vi "Drive_Hardware_Begin.vi"(8 "error in":errorcluster) -> (0 "error out":errorcluster)   [LabVIEW 2020]
uses:
  <vilib>/Rock Robotics/WPI/ThirdParty/Phoenix-LabVIEW/Motor Controller/Controls/CTRE_Phoenix_MotorControl_BaseConfigurables.ctl
  <vilib>/Rock Robotics/WPI/ThirdParty/Phoenix-LabVIEW/Motor Controller/Controls/CTRE_Phoenix_MotorControl_VelocityMeasurementPeriod.ctl
  <vilib>/Rock Robotics/WPI/ThirdParty/Phoenix-LabVIEW/Motor Controller/Controls/CTRE_Phoenix_MotorControl_SlotStructure.ctl
  <vilib>/Rock Robotics/WPI/ThirdParty/Phoenix-LabVIEW/Motor Controller/Controls/CTRE_Phoenix_MotorControl_FilterStruct.ctl
  <vilib>/Rock Robotics/WPI/ThirdParty/Phoenix-LabVIEW/Motor Controller/Controls/CTRE_Phoenix_MotorControl_RemoteSourceType.ctl
  <vilib>/Rock Robotics/WPI/ThirdParty/Phoenix-LabVIEW/Controls/CTRE_Phoenix_CustomParamConfiguration.ctl
  <vilib>/Rock Robotics/WPI/ThirdParty/Phoenix-LabVIEW/Motor Controller/Controls/CTRE_Phoenix_MotorControl_FeedbackDevice_TalonFX.ctl
  <vilib>/Rock Robotics/WPI/ThirdParty/Phoenix-LabVIEW/Motor Controller/Controls/CTRE_Phoenix_MotorControl_LimitSwitchNormal.ctl
  <vilib>/Rock Robotics/WPI/ThirdParty/Phoenix-LabVIEW/Motor Controller/Controls/CTRE_Phoenix_MotorControl_LimitSwitchSource_Local.ctl
  <vilib>/Rock Robotics/WPI/ThirdParty/Phoenix-LabVIEW/Motor Controller/Controls/CTRE_Phoenix_MotorControl_SupplyCurrentLimitConfiguration.ctl
  <vilib>/Rock Robotics/WPI/ThirdParty/Phoenix-LabVIEW/Motor Controller/Controls/CTRE_Phoenix_MotorControl_StatorCurrentLimitConfiguration.ctl
  <vilib>/Rock Robotics/WPI/ThirdParty/Phoenix-LabVIEW/Motor Controller/Controls/CTRE_Phoenix_MotorControl_MotorCommutation_TalonFX.ctl
  <vilib>/Rock Robotics/WPI/ThirdParty/Phoenix-LabVIEW/CANCoder/Controls/CTRE_Phoenix_CANcoder_AbsoluteSensorRange.ctl
  <vilib>/Rock Robotics/WPI/ThirdParty/Phoenix-LabVIEW/CANCoder/Controls/CTRE_Phoenix_CANcoder_SensorInitializationStrategy.ctl
  <vilib>/Rock Robotics/WPI/ThirdParty/Phoenix-LabVIEW/Motor Controller/Controls/CTRE_Phoenix_MotorControl_TalonFXInvertType.ctl
  <vilib>/Rock Robotics/WPI/ThirdParty/Phoenix-LabVIEW/Motor Controller/Controls/CTRE_Phoenix_MotorControl_NeutralMode.ctl
  <vilib>/Rock Robotics/WPI/ThirdParty/Phoenix-LabVIEW/CANCoder/Controls/CTRE_Phoenix_CANcoder_StatusFrame.ctl
  <vilib>/Rock Robotics/WPI/ThirdParty/Phoenix-LabVIEW/Pigeon IMU/CTRE_PigeonIMU_StatusFrameRate.ctl
  Drive_Hardware_Globals.vi
  Globals/Status_Frame_Rate_Globals.vi
  Globals/FilePath_Globals.vi
  Globals/Calibration_And_Constant_Globals.vi
  <vilib>/Utility/file.llb/Read Delimited Spreadsheet (DBL).vi
  Globals/Drive_Globals.vi
panel:
  in  "Front_Right_Zero":dbl[](array[numeric])=[99.4, 331.43]
  in  "Front_Left_Zero":dbl[](array[numeric])=[338.818, 288.54]
  in  "Back_Left_Zero":dbl[](array[numeric])=[255.059, 271.84]
  in  "Back_Right_Zero":dbl[](array[numeric])=[182.197, 189.4]
  out "elements":i32
  out "File Read Error":bool
  out "appended path":path
  in  "Talon FX Configurables":T15={"Base Configurables"={"openLoopRamp"=0.0, "closedLoopRamp"=0.0, "peakOutputForward"=1.0, "peakOutputReverse"=-1.0, "nominalOutputForward"=0.0, "nominalOutputReverse"=0.0, "neutralDeadband"=0.0, "voltageCompSaturation"=0.0, "voltageMeasurementFilter"=32, "velocityMeasurementPeriod"=100, "velocityMeasurementWindow"=64, "forwardSoftLimitThreshold"=0, "reverseSoftLimitThreshold"=0, "forwardSoftLimitEnable"=FALSE, "reverseSoftLimitEnable"=FALSE, "slot0"={"P"=0.0, "I"=0.0, "D"=0.0, "F"=0.0, "integralZone"=0.0, "allowableClosedLoopError"=0, "maxIntegralAccumulator"=0.0, "closedLoopPeakOutput"=1.0, "closedLoopPeriod"=1}, "slot1"={"P"=0.0, "I"=0.0, "D"=0.0, "F"=0.0, "integralZone"=0.0, "allowableClosedLoopError"=0, "maxIntegralAccumulator"=0.0, "closedLoopPeakOutput"=1.0, "closedLoopPeriod"=1}, "slot2"={"P"=0.0, "I"=0.0, "D"=0.0, "F"=0.0, "integralZone"=0.0, "allowableClosedLoopError"=0, "maxIntegralAccumulator"=0.0, "closedLoopPeakOutput"=1.0, "closedLoopPeriod"=1}, "slot3"={"P"=0.0, "I"=0.0, "D"=0.0, "F"=0.0, "integralZone"=0.0, "allowableClosedLoopError"=0, "maxIntegralAccumulator"=0.0, "closedLoopPeakOutput"=1.0, "closedLoopPeriod"=1}, "auxPIDPolarity"=FALSE, "remoteFilter0"={"remoteSensorDeviceID"=0, "remoteSensorSource"=enum."Off"}, "remoteFilter1"={"remoteSensorDeviceID"=0, "remoteSensorSource"=enum."Off"}, "motionCruiseVelocity"=0, "motionAcceleration"=0, "motionProfileTrajectoryPeriod"=0, "feedbackNotContinuous"=FALSE, "remoteSensorClosedLoopDisableNeutralOnLOS"=FALSE, "clearPositionOnLimitF"=FALSE, "clearPositionOnLimitR"=FALSE, "clearPositionOnQuadIdx"=FALSE, "limitSwitchDisableNeutralOnLOS"=FALSE, "softLimitDisableNeutralOnLOS"=FALSE, "pulseWidthPeriod_EdgesPerRot"=1, "pulseWidthPeriod_FilterWindowSz"=1, "customParam"={"customParam0"=0, "customParam1"=0}, "trajectoryInterpolationEnable"=TRUE}, "primaryPID"={"selectedFeedbackCoefficient"=1.0, "selectedFeedbackSensor"=1}, "auxiliaryPID"={"selectedFeedbackCoefficient"=1.0, "selectedFeedbackSensor"=1}, "forwardLimitSwitchNormal"=enum."Normally Open", "reverseLimitSwitchNormal"=enum."Normally Open", "forwardLimitSwitchDeviceID"=0, "reverseLimitSwitchDeviceID"=0, "forwardLimitSwitchSource"=enum."Feedback Connector", "reverseLimitSwitchSource"=enum."Feedback Connector", "sum0Term"=1, "sum1Term"=1, "diff0Term"=1, "diff1Term"=1, "Supply Current Limit Configuration"={"Enable?"=FALSE, "Current Limit"=0.0, "Threshold Current"=0.0, "Threshold Time"=0.0}, "Stator Current Limit Configuration"={"Enable?"=FALSE, "Current Limit"=0.0, "Threshold Current"=0.0, "Threshold Time"=0.0}, "Motor Commutation"=enum."Trapezoidal", "Absolute Sensor Range"=enum."Unsigned [0 to 360)", "Integrated Sensor Offset (Degrees)"=0.0, "Sensor Initialization Strategy"=enum."Boot To Zero"} {"Base Configurables"."velocityMeasurementPeriod" items=["Period_1ms"=1, "Period_2ms"=2, "Period_5ms"=5, "Period_10ms"=10, "Period_20ms"=20, "Period_25ms"=25, "Period_50ms"=50, "Period_100ms"=100]; "primaryPID"."selectedFeedbackSensor" items=["Integrated Sensor"=1, "Sensor Sum (S0 + S1)"=9, "Sensor Difference (D0 - D1)"=10, "Remote Source 0"=11, "Remote Source 1"=12, "None"=14, "Software Emulated"=15]; "auxiliaryPID"."selectedFeedbackSensor" items=["Integrated Sensor"=1, "Sensor Sum (S0 + S1)"=9, "Sensor Difference (D0 - D1)"=10, "Remote Source 0"=11, "Remote Source 1"=12, "None"=14, "Software Emulated"=15]; "sum0Term" items=["Integrated Sensor"=1, "Sensor Sum (S0 + S1)"=9, "Sensor Difference (D0 - D1)"=10, "Remote Source 0"=11, "Remote Source 1"=12, "None"=14, "Software Emulated"=15]; "sum1Term" items=["Integrated Sensor"=1, "Sensor Sum (S0 + S1)"=9, "Sensor Difference (D0 - D1)"=10, "Remote Source 0"=11, "Remote Source 1"=12, "None"=14, "Software Emulated"=15]; "diff0Term" items=["Integrated Sensor"=1, "Sensor Sum (S0 + S1)"=9, "Sensor Difference (D0 - D1)"=10, "Remote Source 0"=11, "Remote Source 1"=12, "None"=14, "Software Emulated"=15]; "diff1Term" items=["Integrated Sensor"=1, "Sensor Sum (S0 + S1)"=9, "Sensor Difference (D0 - D1)"=10, "Remote Source 0"=11, "Remote Source 1"=12, "None"=14, "Software Emulated"=15]}
  # "0th index is alpha, 1st index is beta"
  # "False: Primary Output = PID[0] + PID[1]  ---  Auxiliary Output = PID[0] - PID[1]\nTrue:  Primary Output = PID[0] - PID[1] --- Auxiliary Output = PID[0] + PID[1]"
  # "Enable the motion profile executor to perform linear interpolation between profile points.  Defaults to True."
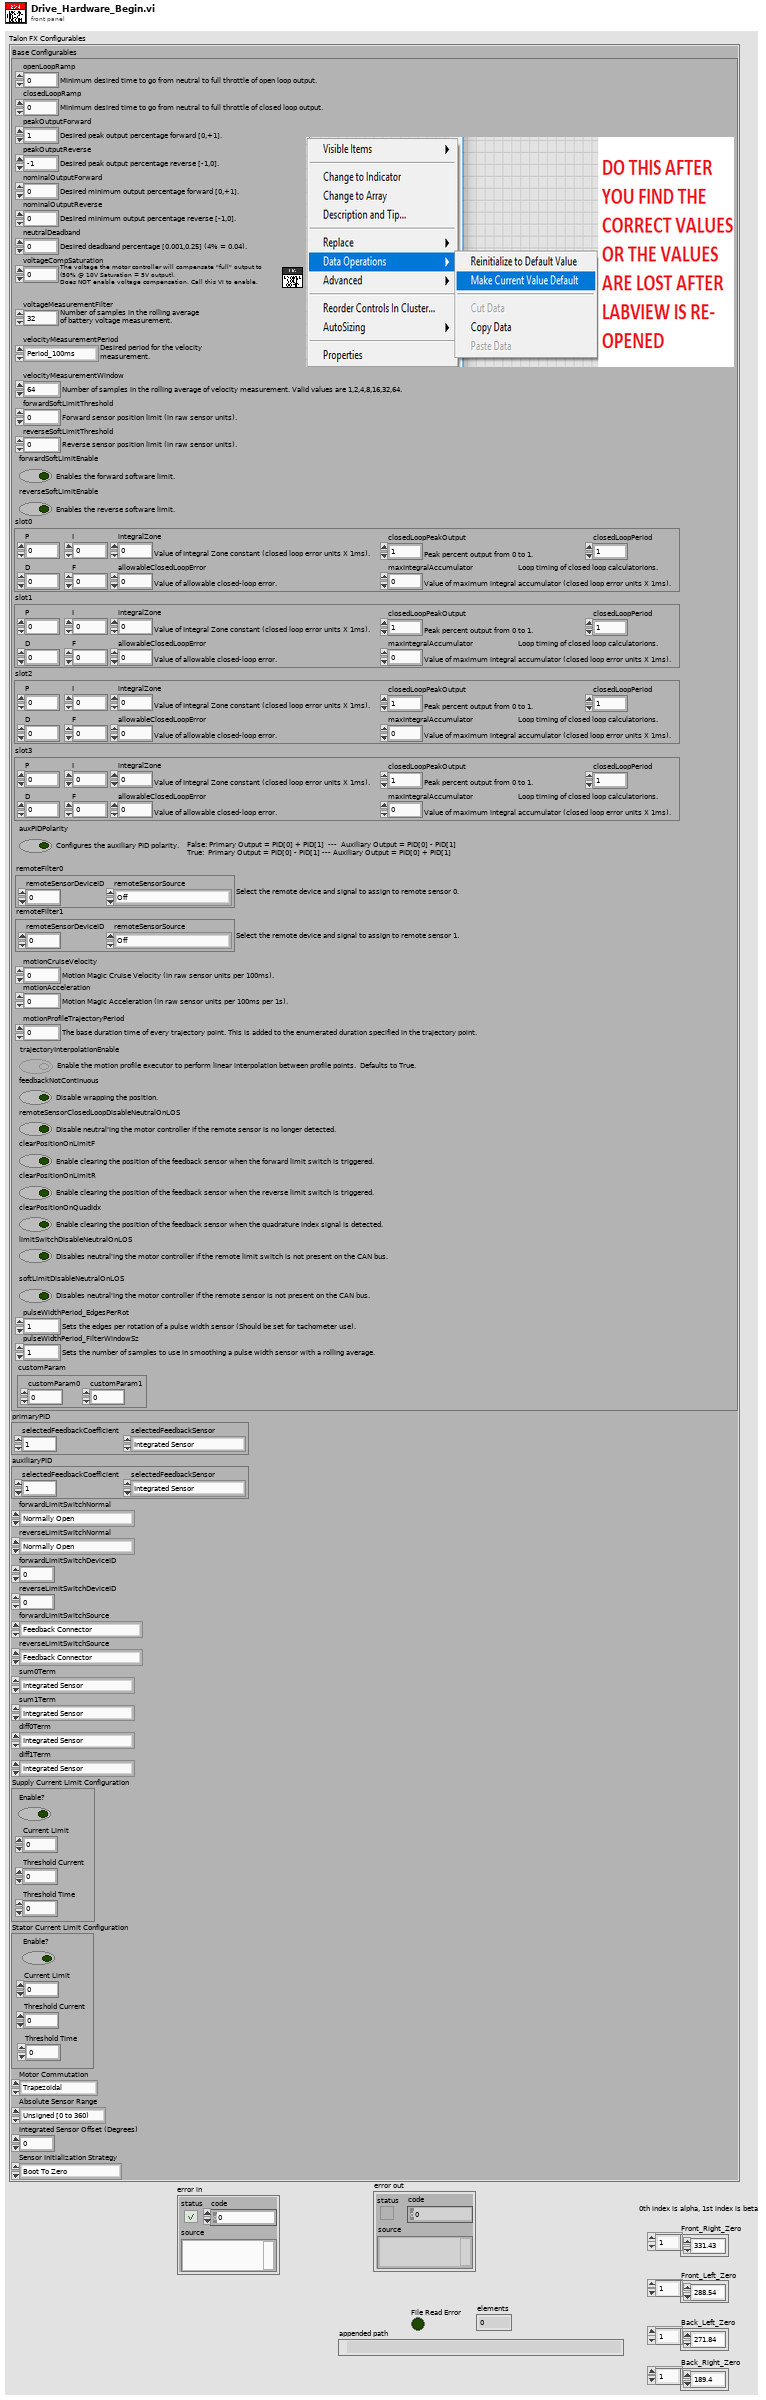
[diagram p1: front panel]
types:
  T1 = typedef "CTRE_Phoenix_MotorControl_BaseConfigurables.ctl" = cluster{"openLoopRamp":dbl, "closedLoopRamp":dbl, "peakOutputForward":dbl, "peakOutputReverse":dbl, "nominalOutputForward":dbl, "nominalOutputReverse":dbl, "neutralDeadband":dbl, "voltageCompSaturation":dbl, "voltageMeasurementFilter":i32, "velocityMeasurementPeriod":T2, "velocityMeasurementWindow":i32, "forwardSoftLimitThreshold":i32, "reverseSoftLimitThreshold":i32, "forwardSoftLimitEnable":bool, "reverseSoftLimitEnable":bool, "slot0":T3, "slot1":T3, "slot2":T3, "slot3":T3, "auxPIDPolarity":bool, "remoteFilter0":T4, "remoteFilter1":T4, "motionCruiseVelocity":i32, "motionAcceleration":i32, "motionProfileTrajectoryPeriod":i32, "feedbackNotContinuous":bool, "remoteSensorClosedLoopDisableNeutralOnLOS":bool, "clearPositionOnLimitF":bool, "clearPositionOnLimitR":bool, "clearPositionOnQuadIdx":bool, "limitSwitchDisableNeutralOnLOS":bool, "softLimitDisableNeutralOnLOS":bool, "pulseWidthPeriod_EdgesPerRot":i32, "pulseWidthPeriod_FilterWindowSz":i32, "customParam":T6, "trajectoryInterpolationEnable":bool}
  T2 = typedef "CTRE_Phoenix_MotorControl_VelocityMeasurementPeriod.ctl" = u16
  T3 = typedef "CTRE_Phoenix_MotorControl_SlotStructure.ctl" = cluster{"P":dbl, "I":dbl, "D":dbl, "F":dbl, "integralZone":dbl, "allowableClosedLoopError":i32, "maxIntegralAccumulator":dbl, "closedLoopPeakOutput":dbl, "closedLoopPeriod":i32}
  T4 = typedef "CTRE_Phoenix_MotorControl_FilterStruct.ctl" = cluster{"remoteSensorDeviceID":u8, "remoteSensorSource":T5}
  T5 = typedef "CTRE_Phoenix_MotorControl_RemoteSourceType.ctl" = enum16{"Off", "Talon SRX Selected Sensor", "Pigeon IMU Yaw", "Pigeon IMU Pitch", "Pigeon IMU Roll", "CANifier Quadrature", "CANifier PWM Input 0", "CANifier PWM Input 1", "CANifier PWM Input 2", "CANifier PWM Input 3", "Gadgeteer Pigeon Yaw", "Gadgeteer Pigeon Pitch", "Gadgeteer Pigeon Roll", "CANCoder"}
  T6 = typedef "CTRE_Phoenix_CustomParamConfiguration.ctl" = cluster{"customParam0":i32, "customParam1":i32}
  T7 = typedef "CTRE_Phoenix_MotorControl_FeedbackDevice_TalonFX.ctl" = i8
  T8 = typedef "CTRE_Phoenix_MotorControl_LimitSwitchNormal.ctl" = enum16{"Normally Open", "Normally Closed", "Disabled"}
  T9 = typedef "CTRE_Phoenix_MotorControl_LimitSwitchSource_Local.ctl" = enum16{"Feedback Connector", "Remote Talon SRX", "Remote CANifier", "Deactivated"}
  T10 = typedef "CTRE_Phoenix_MotorControl_SupplyCurrentLimitConfiguration.ctl" = cluster{"Enable?":bool, "Current Limit":dbl, "Threshold Current":dbl, "Threshold Time":dbl}
  T11 = typedef "CTRE_Phoenix_MotorControl_StatorCurrentLimitConfiguration.ctl" = cluster{"Enable?":bool, "Current Limit":dbl, "Threshold Current":dbl, "Threshold Time":dbl}
  T12 = typedef "CTRE_Phoenix_MotorControl_MotorCommutation_TalonFX.ctl" = enum16{"Trapezoidal"}
  T13 = typedef "CTRE_Phoenix_CANcoder_AbsoluteSensorRange.ctl" = enum16{"Unsigned [0 to 360)", "Signed [-180 to +180)"}
  T14 = typedef "CTRE_Phoenix_CANcoder_SensorInitializationStrategy.ctl" = enum16{"Boot To Zero", "Boot To Absolute Position"}
  T15 = cluster{"Base Configurables":T1, "primaryPID":cluster{"selectedFeedbackCoefficient":dbl, "selectedFeedbackSensor":T7}, "auxiliaryPID":cluster{"selectedFeedbackCoefficient":dbl, "selectedFeedbackSensor":T7}, "forwardLimitSwitchNormal":T8, "reverseLimitSwitchNormal":T8, "forwardLimitSwitchDeviceID":i32, "reverseLimitSwitchDeviceID":i32, "forwardLimitSwitchSource":T9, "reverseLimitSwitchSource":T9, "sum0Term":T7, "sum1Term":T7, "diff0Term":T7, "diff1Term":T7, "Supply Current Limit Configuration":T10, "Stator Current Limit Configuration":T11, "Motor Commutation":T12, "Absolute Sensor Range":T13, "Integrated Sensor Offset (Degrees)":dbl, "Sensor Initialization Strategy":T14}
  T16 = typedef "CTRE_PigeonIMU_StatusFrameRate.ctl" = u32
  T17 = typedef "CTRE_Phoenix_CANcoder_StatusFrame.ctl" = u32
  T18 = typedef "CTRE_Phoenix_MotorControl_TalonFXInvertType.ctl" = enum16{"Counter-Clockwise", "Clockwise"}
  T19 = typedef "CTRE_Phoenix_MotorControl_NeutralMode.ctl" = enum8{"EEPROMSetting", "Override to Coast", "Override to Brake"}
  T20 = typedef "WPI_MotorControlDeviceRef.ctl" = cluster{"DeviceStatus":errorcluster, "Type":T21, "PWM":cluster{"PWM Channel":T22, "DeadBand":T23}, "CAN":cluster{"Device Number":u8, "SetOutput VI Ref":variant, "GetOutput VI Ref":variant, "Enable VI Ref":variant, "Disable VI Ref":variant, "Data":variant}, "Invert":bool, "DIO PWM":cluster{"PWM \"Enable\" Channel":T22, "DIOChannel":T24, "PWM Rate":dbl}}
  T21 = typedef "WPI_MotorControlType.ctl" = enum16{"PWM", "CAN", "DIO PWM"}
  T22 = typedef "FPGA_DIOPWMChannel.ctl" = enum8{"PWM 0", "PWM 1", "PWM 2", "PWM 3", "PWM 4", "PWM 5", "PWM 6", "PWM 7", "PWM 8", "PWM 9", "PWM MXP 0", "PWM MXP 1", "PWM MXP 2", "PWM MXP 3", "PWM MXP 4", "PWM MXP 5", "PWM MXP 6", "PWM MXP 7", "PWM MXP 8", "PWM MXP 9", "Invalid"}
  T23 = typedef "WPI_PWMDeadband.ctl" = cluster{"Name":string, "maxPositivePwm":i32, "minPositivePwm":i32, "centerPwm":i32, "maxNegativePwm":i32, "minNegativePwm":i32, "angularRange":u16}
  T24 = typedef "FPGA_DIOChannel.ctl" = enum8{"DIO 0", "DIO 1", "DIO 2", "DIO 3", "DIO 4", "DIO 5", "DIO 6", "DIO 7", "DIO 8", "DIO 9", "DIO MXP 0", "DIO MXP 1", "DIO MXP 2", "DIO MXP 3", "DIO MXP 4", "DIO MXP 5", "DIO MXP 6", "DIO MXP 7", "DIO MXP 8", "DIO MXP 9", "DIO MXP 10", "DIO MXP 11", "DIO MXP 12", "DIO MXP 13", "DIO MXP 14", "DIO MXP 15", "SPI Port CS1", "SPI Port CS2", "SPI Port CS3", "SPI Port MISO", "SPI Port MOSI", "Invalid"}
  T25 = typedef "CTRE_PigeonIMU_DeviceRef.ctl" = cluster{"DeviceStatus":errorcluster, "Device Number":u8, "Type":T26, "Device ID":u32, "Handle":u64, "UsageFrame":u32, "Library Path":path}
  T26 = typedef "CTRE_PigeonIMU_ConnectionType.ctl" = u32
  T27 = typedef "CTRE_Phoenix_CANcoder_DeviceRef.ctl" = cluster{"DeviceStatus":errorcluster, "Device Number":u8, "Handle":u64, "UsageFrame":u32, "Library Path":path}
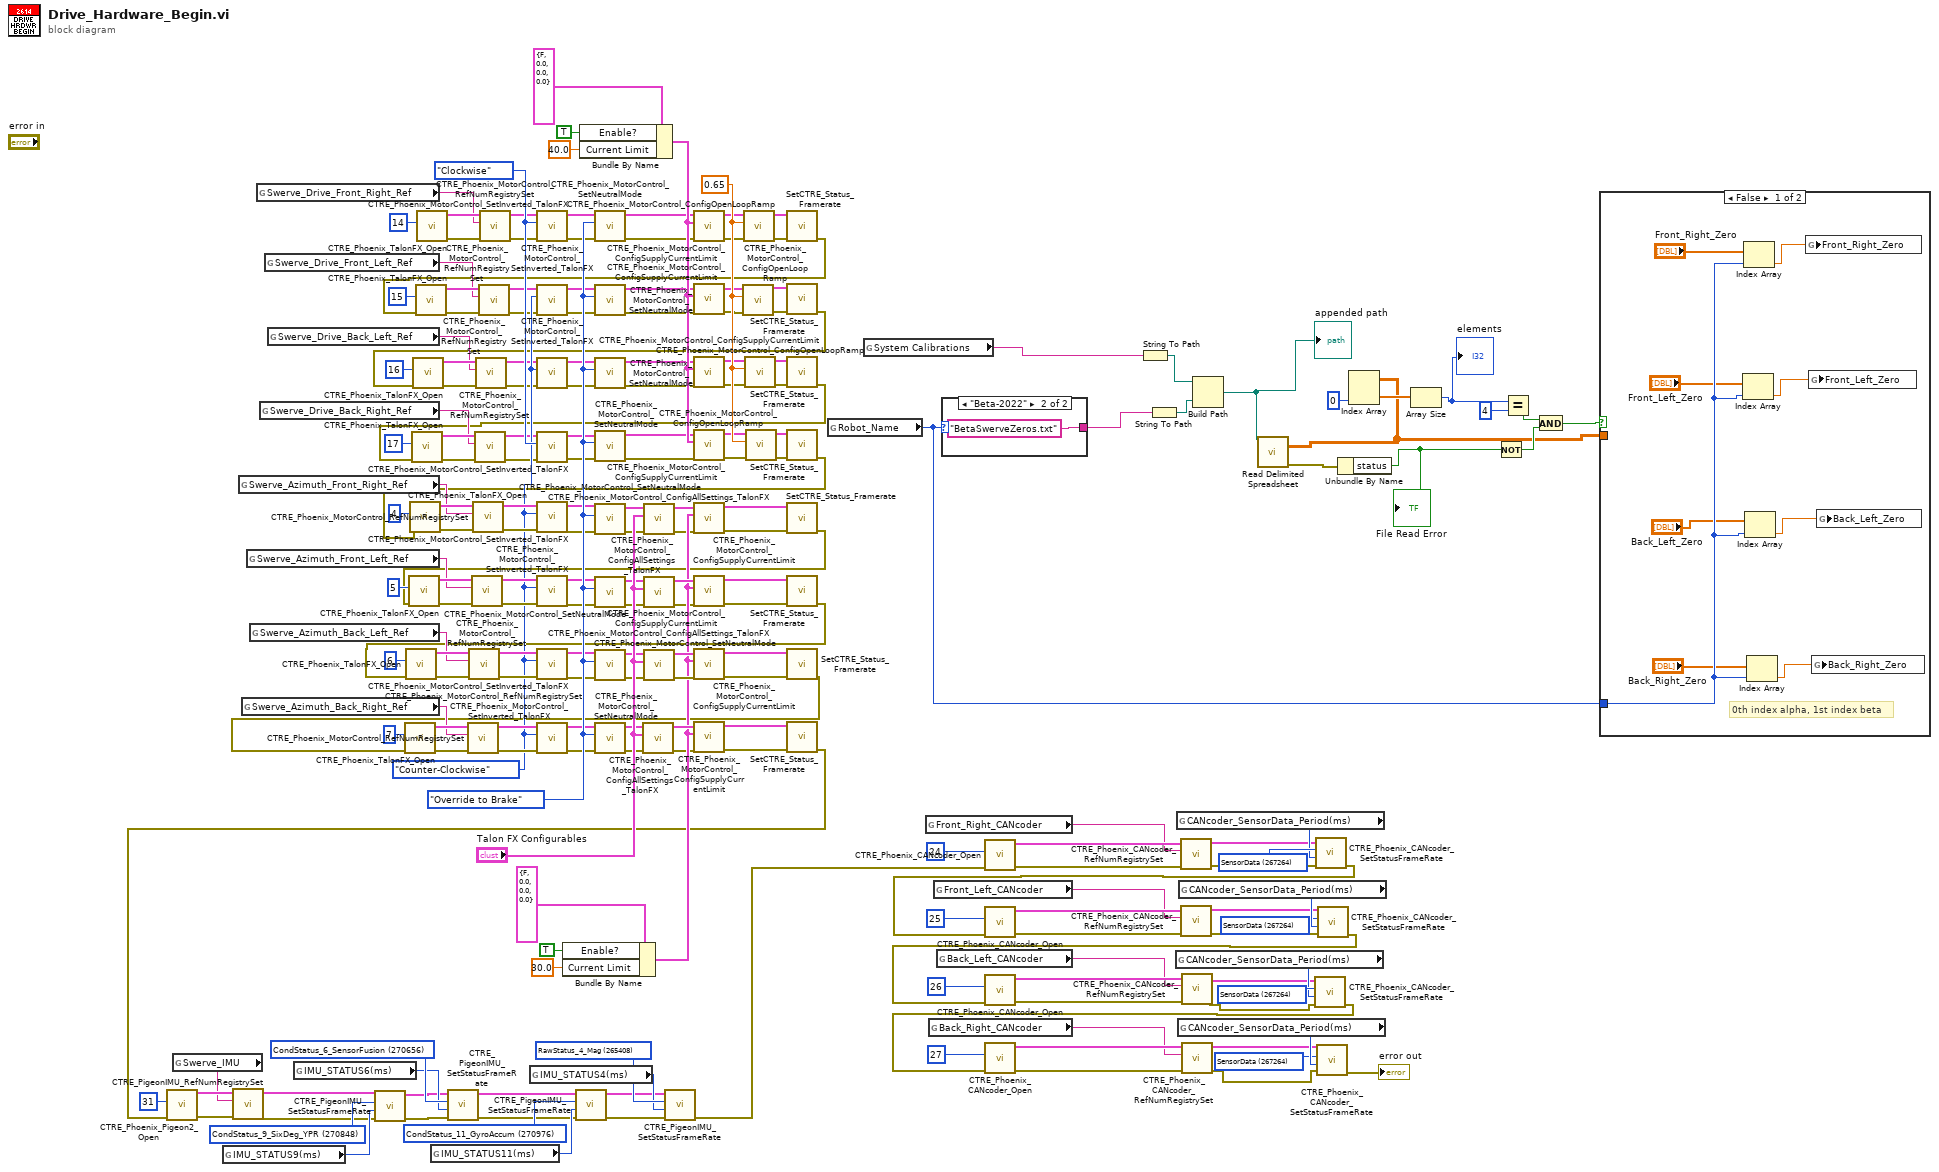
[diagram p0: block diagram]
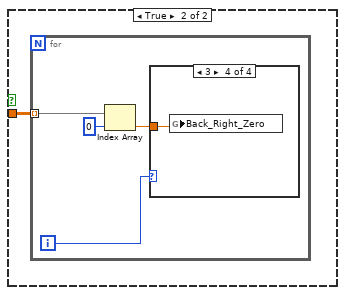
[diagram p2: hidden frame]
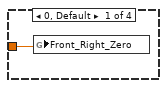
[diagram p3: hidden frame]
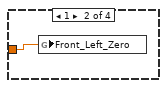
[diagram p4: hidden frame]
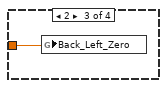
[diagram p5: hidden frame]
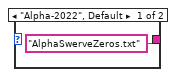
[diagram p6: hidden frame]
diagram:
  w31 = T16 265408 items=["CondStatus_1_General"=270336, "CondStatus_9_SixDeg_YPR"=270848, "CondStatus_6_SensorFusion"=270656, "CondStatus_11_GyroAccum"=270976, "CondStatus_2_GeneralCompass"=270400, "CondStatus_3_GeneralAccel"=270464, "CondStatus_10_SixDeg_Quat"=270912, "RawStatus_4_Mag"=265408, "BiasedStatus_2_Gyro"=269376, "BiasedStatus_4_Mag"=269504, "BiasedStatus_6_Accel"=269632] ("Pigeon IMU Status Frame")
  w32 = T16 270976 items=["CondStatus_1_General"=270336, "CondStatus_9_SixDeg_YPR"=270848, "CondStatus_6_SensorFusion"=270656, "CondStatus_11_GyroAccum"=270976, "CondStatus_2_GeneralCompass"=270400, "CondStatus_3_GeneralAccel"=270464, "CondStatus_10_SixDeg_Quat"=270912, "RawStatus_4_Mag"=265408, "BiasedStatus_2_Gyro"=269376, "BiasedStatus_4_Mag"=269504, "BiasedStatus_6_Accel"=269632] ("Pigeon IMU Status Frame")
  w33 = T16 270656 items=["CondStatus_1_General"=270336, "CondStatus_9_SixDeg_YPR"=270848, "CondStatus_6_SensorFusion"=270656, "CondStatus_11_GyroAccum"=270976, "CondStatus_2_GeneralCompass"=270400, "CondStatus_3_GeneralAccel"=270464, "CondStatus_10_SixDeg_Quat"=270912, "RawStatus_4_Mag"=265408, "BiasedStatus_2_Gyro"=269376, "BiasedStatus_4_Mag"=269504, "BiasedStatus_6_Accel"=269632] ("Pigeon IMU Status Frame")
  w34 = T16 270848 items=["CondStatus_1_General"=270336, "CondStatus_9_SixDeg_YPR"=270848, "CondStatus_6_SensorFusion"=270656, "CondStatus_11_GyroAccum"=270976, "CondStatus_2_GeneralCompass"=270400, "CondStatus_3_GeneralAccel"=270464, "CondStatus_10_SixDeg_Quat"=270912, "RawStatus_4_Mag"=265408, "BiasedStatus_2_Gyro"=269376, "BiasedStatus_4_Mag"=269504, "BiasedStatus_6_Accel"=269632] ("Pigeon IMU Status Frame")
  w45 = T17 267264 items=["SensorData"=267264, "VbatAndFaults"=267328] ("CANcoder Status Frame")
  w48 = T17 267264 items=["SensorData"=267264, "VbatAndFaults"=267328] ("CANcoder Status Frame")
  w49 = T17 267264 items=["SensorData"=267264, "VbatAndFaults"=267328] ("CANcoder Status Frame")
  w54 = T17 267264 items=["SensorData"=267264, "VbatAndFaults"=267328] ("CANcoder Status Frame")
  w131 = 0.65 ("secondsFromNeutralToFull")
  w149 = CTRE_Phoenix_MotorControl_TalonFXInvertType."Clockwise" ("Invert Type")
  w197 = CTRE_Phoenix_MotorControl_NeutralMode."Override to Brake" ("Motor Control Neutral Mode")
  w148 = CTRE_Phoenix_MotorControl_TalonFXInvertType."Counter-Clockwise" ("Invert Type")
  n1 = global read "Drive_Hardware_Globals.vi" "Swerve_IMU"() -> (w128:string)
  n2 = global read "Status_Frame_Rate_Globals.vi" "IMU_STATUS9(ms)"() -> (w30:i16)
  n3 = global read "Drive_Hardware_Globals.vi" "Swerve_Azimuth_Front_Right_Ref"() -> (w169:string)
  n4 = global read "Drive_Hardware_Globals.vi" "Swerve_Azimuth_Back_Right_Ref"() -> (w166:string)
  n5 = global read "Drive_Hardware_Globals.vi" "Swerve_Azimuth_Front_Left_Ref"() -> (w168:string)
  n6 = global read "Drive_Hardware_Globals.vi" "Swerve_Azimuth_Back_Left_Ref"() -> (w167:string)
  n7 = global read "Drive_Hardware_Globals.vi" "Swerve_Drive_Front_Right_Ref"() -> (w119:string)
  n8 = global read "Drive_Hardware_Globals.vi" "Swerve_Drive_Back_Right_Ref"() -> (w83:string)
  n9 = global read "Drive_Hardware_Globals.vi" "Swerve_Drive_Front_Left_Ref"() -> (w107:string)
  n10 = global read "Drive_Hardware_Globals.vi" "Swerve_Drive_Back_Left_Ref"() -> (w95:string)
  n11 = global read "Status_Frame_Rate_Globals.vi" "IMU_STATUS6(ms)"() -> (w29:i16)
  n12 = call <vilib>:"CTRE_Phoenix_TalonFX_Open.vi"("Device Number"=u8 14) -> ("error out"=w123:errorcluster, "PhoenixMotorControlDevRef"=w120:T20)  [unwired: 9 in]
  n13 = global read "Status_Frame_Rate_Globals.vi" "IMU_STATUS11(ms)"() -> (w28:i16)
  n14 = call <vilib>:"CTRE_Phoenix_MotorControl_RefNumRegistrySet.vi"("error in (no error)"=w123, "refnum name"=w119, "PhoenixMotorControlDevRef"=w120) -> ("error out"=w122:errorcluster, "PhoenixMotorControlDevRef"=w121:T20)  [unwired: 7 in]
  n15 = global read "Status_Frame_Rate_Globals.vi" "IMU_STATUS4(ms)"() -> (w27:i16)
  n16 = call <vilib>:"CTRE_Phoenix_MotorControl_SetInverted_TalonFX.vi"("error in (no error)"=w122, "Invert Type"=w149, "PhoenixMotorControlDevRef"=w121) -> ("error out"=w126:errorcluster, "PhoenixMotorControlDevRef"=w125:T20)  [unwired: 7 in]
  n17 = Bundle By Name(cluster=T10 {"Enable?"=FALSE, "Current Limit"=0.0, "Threshold Current"=0.0, "Threshold Time"=0.0} ("Supply Current Limit Configuration"), "Enable?"=TRUE, "Current Limit"=30.0) -> (w157:T10)
  n18 = Bundle By Name(cluster=T10 {"Enable?"=FALSE, "Current Limit"=0.0, "Threshold Current"=0.0, "Threshold Time"=0.0} ("Supply Current Limit Configuration"), "Enable?"=TRUE, "Current Limit"=40.0) -> (w150:T10)
  n19 = call <vilib>:"CTRE_Phoenix_MotorControl_SetNeutralMode.vi"("error in (no error)"=w126, "Motor Control Neutral Mode"=w197, "PhoenixMotorControlDevRef"=w125) -> ("error out"=w117:errorcluster, "PhoenixMotorControlDevRef"=w118:T20)  [unwired: 7 in]
  n20 = call <vilib>:"CTRE_Phoenix_MotorControl_ConfigSupplyCurrentLimit.vi"("error in (no error)"=w117, "Supply Current Limit Configuration"=w150, "PhoenixMotorControlDevRef"=w118) -> ("error out"=w116:errorcluster, "PhoenixMotorControlDevRef"=w115:T20)  [unwired: 7 in]
  n21 = call <vilib>:"CTRE_Phoenix_MotorControl_ConfigOpenLoopRamp.vi"("error in (no error)"=w116, "secondsFromNeutralToFull"=w131, "PhoenixMotorControlDevRef"=w115) -> ("error out"=w73:errorcluster, "PhoenixMotorControlDevRef"=w74:T20)  [unwired: 7 in]
  n22 = call "SetCTRE_Status_Framerate.vi"("error in (no error)"=w73, "PhoenixMotorControlDevRef"=w74) -> ("error out"=w63:errorcluster)  [unwired: 8 in, 1 out]
  n23 = call <vilib>:"CTRE_Phoenix_TalonFX_Open.vi"("error in"=w63, "Device Number"=u8 15) -> ("error out"=w109:errorcluster, "PhoenixMotorControlDevRef"=w112:T20)  [unwired: 8 in]
  n24 = call <vilib>:"CTRE_Phoenix_MotorControl_RefNumRegistrySet.vi"("error in (no error)"=w109, "refnum name"=w107, "PhoenixMotorControlDevRef"=w112) -> ("error out"=w110:errorcluster, "PhoenixMotorControlDevRef"=w111:T20)  [unwired: 7 in]
  n25 = call <vilib>:"CTRE_Phoenix_MotorControl_SetInverted_TalonFX.vi"("error in (no error)"=w110, "Invert Type"=w148, "PhoenixMotorControlDevRef"=w111) -> ("error out"=w114:errorcluster, "PhoenixMotorControlDevRef"=w113:T20)  [unwired: 7 in]
  n26 = call <vilib>:"CTRE_Phoenix_MotorControl_SetNeutralMode.vi"("error in (no error)"=w114, "Motor Control Neutral Mode"=w197, "PhoenixMotorControlDevRef"=w113) -> ("error out"=w105:errorcluster, "PhoenixMotorControlDevRef"=w106:T20)  [unwired: 7 in]
  n27 = call <vilib>:"CTRE_Phoenix_MotorControl_ConfigSupplyCurrentLimit.vi"("error in (no error)"=w105, "Supply Current Limit Configuration"=w150, "PhoenixMotorControlDevRef"=w106) -> ("error out"=w104:errorcluster, "PhoenixMotorControlDevRef"=w103:T20)  [unwired: 7 in]
  n28 = call <vilib>:"CTRE_Phoenix_MotorControl_ConfigOpenLoopRamp.vi"("error in (no error)"=w104, "secondsFromNeutralToFull"=w131, "PhoenixMotorControlDevRef"=w103) -> ("error out"=w71:errorcluster, "PhoenixMotorControlDevRef"=w72:T20)  [unwired: 7 in]
  n29 = call "SetCTRE_Status_Framerate.vi"("error in (no error)"=w71, "PhoenixMotorControlDevRef"=w72) -> ("error out"=w62:errorcluster)  [unwired: 8 in, 1 out]
  n30 = call <vilib>:"CTRE_Phoenix_TalonFX_Open.vi"("error in"=w62, "Device Number"=u8 16) -> ("error out"=w97:errorcluster, "PhoenixMotorControlDevRef"=w100:T20)  [unwired: 8 in]
  n31 = call <vilib>:"CTRE_Phoenix_MotorControl_RefNumRegistrySet.vi"("error in (no error)"=w97, "refnum name"=w95, "PhoenixMotorControlDevRef"=w100) -> ("error out"=w98:errorcluster, "PhoenixMotorControlDevRef"=w99:T20)  [unwired: 7 in]
  n32 = call <vilib>:"CTRE_Phoenix_MotorControl_SetInverted_TalonFX.vi"("error in (no error)"=w98, "Invert Type"=w148, "PhoenixMotorControlDevRef"=w99) -> ("error out"=w102:errorcluster, "PhoenixMotorControlDevRef"=w101:T20)  [unwired: 7 in]
  n33 = call <vilib>:"CTRE_Phoenix_MotorControl_SetNeutralMode.vi"("error in (no error)"=w102, "Motor Control Neutral Mode"=w197, "PhoenixMotorControlDevRef"=w101) -> ("error out"=w93:errorcluster, "PhoenixMotorControlDevRef"=w94:T20)  [unwired: 7 in]
  n34 = call <vilib>:"CTRE_Phoenix_MotorControl_ConfigSupplyCurrentLimit.vi"("error in (no error)"=w93, "Supply Current Limit Configuration"=w150, "PhoenixMotorControlDevRef"=w94) -> ("error out"=w92:errorcluster, "PhoenixMotorControlDevRef"=w91:T20)  [unwired: 7 in]
  n35 = call <vilib>:"CTRE_Phoenix_MotorControl_ConfigOpenLoopRamp.vi"("error in (no error)"=w92, "secondsFromNeutralToFull"=w131, "PhoenixMotorControlDevRef"=w91) -> ("error out"=w69:errorcluster, "PhoenixMotorControlDevRef"=w70:T20)  [unwired: 7 in]
  n36 = call "SetCTRE_Status_Framerate.vi"("error in (no error)"=w69, "PhoenixMotorControlDevRef"=w70) -> ("error out"=w61:errorcluster)  [unwired: 8 in, 1 out]
  n37 = call <vilib>:"CTRE_Phoenix_TalonFX_Open.vi"("error in"=w61, "Device Number"=u8 17) -> ("error out"=w87:errorcluster, "PhoenixMotorControlDevRef"=w84:T20)  [unwired: 8 in]
  n38 = call <vilib>:"CTRE_Phoenix_MotorControl_RefNumRegistrySet.vi"("error in (no error)"=w87, "refnum name"=w83, "PhoenixMotorControlDevRef"=w84) -> ("error out"=w86:errorcluster, "PhoenixMotorControlDevRef"=w85:T20)  [unwired: 7 in]
  n39 = call <vilib>:"CTRE_Phoenix_MotorControl_SetInverted_TalonFX.vi"("error in (no error)"=w86, "Invert Type"=w149, "PhoenixMotorControlDevRef"=w85) -> ("error out"=w90:errorcluster, "PhoenixMotorControlDevRef"=w89:T20)  [unwired: 7 in]
  n40 = call <vilib>:"CTRE_Phoenix_MotorControl_SetNeutralMode.vi"("error in (no error)"=w90, "Motor Control Neutral Mode"=w197, "PhoenixMotorControlDevRef"=w89) -> ("error out"=w81:errorcluster, "PhoenixMotorControlDevRef"=w82:T20)  [unwired: 7 in]
  n41 = call <vilib>:"CTRE_Phoenix_MotorControl_ConfigSupplyCurrentLimit.vi"("error in (no error)"=w81, "Supply Current Limit Configuration"=w150, "PhoenixMotorControlDevRef"=w82) -> ("error out"=w79:errorcluster, "PhoenixMotorControlDevRef"=w80:T20)  [unwired: 7 in]
  n42 = call <vilib>:"CTRE_Phoenix_MotorControl_ConfigOpenLoopRamp.vi"("error in (no error)"=w79, "secondsFromNeutralToFull"=w131, "PhoenixMotorControlDevRef"=w80) -> ("error out"=w78:errorcluster, "PhoenixMotorControlDevRef"=w77:T20)  [unwired: 7 in]
  n43 = call "SetCTRE_Status_Framerate.vi"("error in (no error)"=w78, "PhoenixMotorControlDevRef"=w77) -> ("error out"=w60:errorcluster)  [unwired: 8 in, 1 out]
  n44 = call <vilib>:"CTRE_Phoenix_TalonFX_Open.vi"("error in"=w60, "Device Number"=u8 4) -> ("error out"=w185:errorcluster, "PhoenixMotorControlDevRef"=w188:T20)  [unwired: 8 in]
  n45 = call <vilib>:"CTRE_Phoenix_MotorControl_RefNumRegistrySet.vi"("error in (no error)"=w185, "refnum name"=w169, "PhoenixMotorControlDevRef"=w188) -> ("error out"=w186:errorcluster, "PhoenixMotorControlDevRef"=w187:T20)  [unwired: 7 in]
  n46 = call <vilib>:"CTRE_Phoenix_MotorControl_SetInverted_TalonFX.vi"("error in (no error)"=w186, "Invert Type"=w148, "PhoenixMotorControlDevRef"=w187) -> ("error out"=w192:errorcluster, "PhoenixMotorControlDevRef"=w191:T20)  [unwired: 7 in]
  n47 = call <vilib>:"CTRE_Phoenix_MotorControl_SetNeutralMode.vi"("error in (no error)"=w192, "Motor Control Neutral Mode"=w197, "PhoenixMotorControlDevRef"=w191) -> ("error out"=w204:errorcluster, "PhoenixMotorControlDevRef"=w205:T20)  [unwired: 7 in]
  n48 = call <vilib>:"CTRE_Phoenix_MotorControl_ConfigAllSettings_TalonFX.vi"("error in (no error)"=w204, "Talon FX Configurables"="Talon FX Configurables", "PhoenixMotorControlDevRef"=w205) -> ("error out"=w156:errorcluster, "PhoenixMotorControlDevRef"=w163:T20)  [unwired: 7 in]
  n49 = call <vilib>:"CTRE_Phoenix_MotorControl_ConfigSupplyCurrentLimit.vi"("error in (no error)"=w156, "Supply Current Limit Configuration"=w157, "PhoenixMotorControlDevRef"=w163) -> ("error out"=w68:errorcluster, "PhoenixMotorControlDevRef"=w17:T20)  [unwired: 7 in]
  n50 = call "SetCTRE_Status_Framerate.vi"("error in (no error)"=w68, "PhoenixMotorControlDevRef"=w17) -> ("error out"=w59:errorcluster)  [unwired: 8 in, 1 out]
  n51 = call <vilib>:"CTRE_Phoenix_TalonFX_Open.vi"("error in"=w59, "Device Number"=u8 5) -> ("error out"=w182:errorcluster, "PhoenixMotorControlDevRef"=w179:T20)  [unwired: 8 in]
  n52 = call <vilib>:"CTRE_Phoenix_MotorControl_RefNumRegistrySet.vi"("error in (no error)"=w182, "refnum name"=w168, "PhoenixMotorControlDevRef"=w179) -> ("error out"=w181:errorcluster, "PhoenixMotorControlDevRef"=w180:T20)  [unwired: 7 in]
  n53 = call <vilib>:"CTRE_Phoenix_MotorControl_SetInverted_TalonFX.vi"("error in (no error)"=w181, "Invert Type"=w148, "PhoenixMotorControlDevRef"=w180) -> ("error out"=w194:errorcluster, "PhoenixMotorControlDevRef"=w193:T20)  [unwired: 7 in]
  n54 = call <vilib>:"CTRE_Phoenix_MotorControl_SetNeutralMode.vi"("error in (no error)"=w194, "Motor Control Neutral Mode"=w197, "PhoenixMotorControlDevRef"=w193) -> ("error out"=w202:errorcluster, "PhoenixMotorControlDevRef"=w203:T20)  [unwired: 7 in]
  n55 = call <vilib>:"CTRE_Phoenix_MotorControl_ConfigAllSettings_TalonFX.vi"("error in (no error)"=w202, "Talon FX Configurables"="Talon FX Configurables", "PhoenixMotorControlDevRef"=w203) -> ("error out"=w155:errorcluster, "PhoenixMotorControlDevRef"=w162:T20)  [unwired: 7 in]
  n56 = call <vilib>:"CTRE_Phoenix_MotorControl_ConfigSupplyCurrentLimit.vi"("error in (no error)"=w155, "Supply Current Limit Configuration"=w157, "PhoenixMotorControlDevRef"=w162) -> ("error out"=w66:errorcluster, "PhoenixMotorControlDevRef"=w67:T20)  [unwired: 7 in]
  n57 = call "SetCTRE_Status_Framerate.vi"("error in (no error)"=w66, "PhoenixMotorControlDevRef"=w67) -> ("error out"=w58:errorcluster)  [unwired: 8 in, 1 out]
  n58 = call <vilib>:"CTRE_Phoenix_TalonFX_Open.vi"("error in"=w58, "Device Number"=u8 6) -> ("error out"=w57:errorcluster, "PhoenixMotorControlDevRef"=w170:T20)  [unwired: 8 in]
  n59 = call <vilib>:"CTRE_Phoenix_MotorControl_RefNumRegistrySet.vi"("error in (no error)"=w57, "refnum name"=w167, "PhoenixMotorControlDevRef"=w170) -> ("error out"=w172:errorcluster, "PhoenixMotorControlDevRef"=w171:T20)  [unwired: 7 in]
  n60 = call <vilib>:"CTRE_Phoenix_MotorControl_SetInverted_TalonFX.vi"("error in (no error)"=w172, "Invert Type"=w148, "PhoenixMotorControlDevRef"=w171) -> ("error out"=w196:errorcluster, "PhoenixMotorControlDevRef"=w195:T20)  [unwired: 7 in]
  n61 = call <vilib>:"CTRE_Phoenix_MotorControl_SetNeutralMode.vi"("error in (no error)"=w196, "Motor Control Neutral Mode"=w197, "PhoenixMotorControlDevRef"=w195) -> ("error out"=w201:errorcluster, "PhoenixMotorControlDevRef"=w200:T20)  [unwired: 7 in]
  n62 = call <vilib>:"CTRE_Phoenix_MotorControl_ConfigAllSettings_TalonFX.vi"("error in (no error)"=w201, "Talon FX Configurables"="Talon FX Configurables", "PhoenixMotorControlDevRef"=w200) -> ("error out"=w165:errorcluster, "PhoenixMotorControlDevRef"=w164:T20)  [unwired: 7 in]
  n63 = call <vilib>:"CTRE_Phoenix_MotorControl_ConfigSupplyCurrentLimit.vi"("error in (no error)"=w165, "Supply Current Limit Configuration"=w157, "PhoenixMotorControlDevRef"=w164) -> ("error out"=w64:errorcluster, "PhoenixMotorControlDevRef"=w65:T20)  [unwired: 7 in]
  n64 = call "SetCTRE_Status_Framerate.vi"("error in (no error)"=w64, "PhoenixMotorControlDevRef"=w65) -> ("error out"=w56:errorcluster)  [unwired: 8 in, 1 out]
  n65 = call <vilib>:"CTRE_Phoenix_TalonFX_Open.vi"("error in"=w56, "Device Number"=u8 7) -> ("error out"=w175:errorcluster, "PhoenixMotorControlDevRef"=w178:T20)  [unwired: 8 in]
  n66 = call <vilib>:"CTRE_Phoenix_MotorControl_RefNumRegistrySet.vi"("error in (no error)"=w175, "refnum name"=w166, "PhoenixMotorControlDevRef"=w178) -> ("error out"=w176:errorcluster, "PhoenixMotorControlDevRef"=w177:T20)  [unwired: 7 in]
  n67 = call <vilib>:"CTRE_Phoenix_MotorControl_SetInverted_TalonFX.vi"("error in (no error)"=w176, "Invert Type"=w148, "PhoenixMotorControlDevRef"=w177) -> ("error out"=w190:errorcluster, "PhoenixMotorControlDevRef"=w189:T20)  [unwired: 7 in]
  n68 = call <vilib>:"CTRE_Phoenix_MotorControl_SetNeutralMode.vi"("error in (no error)"=w190, "Motor Control Neutral Mode"=w197, "PhoenixMotorControlDevRef"=w189) -> ("error out"=w199:errorcluster, "PhoenixMotorControlDevRef"=w198:T20)  [unwired: 7 in]
  n69 = call <vilib>:"CTRE_Phoenix_MotorControl_ConfigAllSettings_TalonFX.vi"("error in (no error)"=w199, "Talon FX Configurables"="Talon FX Configurables", "PhoenixMotorControlDevRef"=w198) -> ("error out"=w154:errorcluster, "PhoenixMotorControlDevRef"=w161:T20)  [unwired: 7 in]
  n70 = call <vilib>:"CTRE_Phoenix_MotorControl_ConfigSupplyCurrentLimit.vi"("error in (no error)"=w154, "Supply Current Limit Configuration"=w157, "PhoenixMotorControlDevRef"=w161) -> ("error out"=w75:errorcluster, "PhoenixMotorControlDevRef"=w76:T20)  [unwired: 7 in]
  n71 = call "SetCTRE_Status_Framerate.vi"("error in (no error)"=w75, "PhoenixMotorControlDevRef"=w76) -> ("error out"=w55:errorcluster)  [unwired: 8 in, 1 out]
  n72 = call <vilib>:"CTRE_Phoenix_Pigeon2_Open.vi"("error in"=w55, "Device Number"=u8 31) -> ("error out"=w129:errorcluster, "PigeonIMUDevRef"=w130:T25)  [unwired: 8 in]
  n73 = call <vilib>:"CTRE_PigeonIMU_RefNumRegistrySet.vi"("error in (no error)"=w129, "refnum name"=w128, "PigeonIMUDevRef"=w130) -> ("error out"=w19:errorcluster, "PigeonIMUDevRef"=w20:T25)  [unwired: 7 in]
  n74 = call <vilib>:"CTRE_PigeonIMU_SetStatusFrameRate.vi"("error in (no error)"=w19, "Period (ms)"=w30, "StatusFrame"=w34, "PigeonIMUDevRef"=w20) -> ("error out"=w25:errorcluster, "PigeonIMUDevRef"=w26:T25)  [unwired: 6 in]
  n75 = call <vilib>:"CTRE_PigeonIMU_SetStatusFrameRate.vi"("error in (no error)"=w25, "Period (ms)"=w29, "StatusFrame"=w33, "PigeonIMUDevRef"=w26) -> ("error out"=w23:errorcluster, "PigeonIMUDevRef"=w24:T25)  [unwired: 6 in]
  n76 = call <vilib>:"CTRE_PigeonIMU_SetStatusFrameRate.vi"("error in (no error)"=w23, "Period (ms)"=w28, "StatusFrame"=w32, "PigeonIMUDevRef"=w24) -> ("error out"=w21:errorcluster, "PigeonIMUDevRef"=w22:T25)  [unwired: 6 in]
  n77 = call <vilib>:"CTRE_PigeonIMU_SetStatusFrameRate.vi"("error in (no error)"=w21, "Period (ms)"=w27, "StatusFrame"=w31, "PigeonIMUDevRef"=w22) -> ("error out"=w18:errorcluster)  [unwired: 6 in, 1 out]
  n78 = global read "Calibration_And_Constant_Globals.vi" "Robot_Name"() -> (w1:enum16{"Alpha-2022", "Beta-2022"})
  n79 = global read "FilePath_Globals.vi" "System Calibrations"() -> (w5:string)
  n80 = global read "Drive_Hardware_Globals.vi" "Front_Right_CANcoder"() -> (w135:string)
  n81 = global read "Drive_Hardware_Globals.vi" "Back_Right_CANcoder"() -> (w132:string)
  n82 = global read "Drive_Hardware_Globals.vi" "Front_Left_CANcoder"() -> (w134:string)
  n83 = global read "Drive_Hardware_Globals.vi" "Back_Left_CANcoder"() -> (w133:string)
  n84 = case shown="\"Beta-2022\"" w1 {
    tunnel: ["AlphaSwerveZeros.txt" ("string") "BetaSwerveZeros.txt" ("string")] -> w4
    frame "Alpha-2022", Default {
    }
    frame "Beta-2022" {
    }
  }
  n85 = call <vilib>:"CTRE_Phoenix_CANcoder_Open.vi"("error in"=w18, "Device Number"=u8 24) -> ("error out"=w142:errorcluster, "CTRE_CANcoder_DeviceRef"=w143:T27)  [unwired: 8 in]
  n86 = String To Path(string=w5) -> (path=w16:path)
  n87 = String To Path(string=w4) -> (path=w8:path)
  n88 = global read "Status_Frame_Rate_Globals.vi" "CANcoder_SensorData_Period(ms)"() -> (w47:u8)
  n89 = global read "Status_Frame_Rate_Globals.vi" "CANcoder_SensorData_Period(ms)"() -> (w53:u8)
  n90 = global read "Status_Frame_Rate_Globals.vi" "CANcoder_SensorData_Period(ms)"() -> (w46:u8)
  n91 = global read "Status_Frame_Rate_Globals.vi" "CANcoder_SensorData_Period(ms)"() -> (w50:u8)
  n92 = call <vilib>:"CTRE_Phoenix_CANcoder_RefNumRegistrySet.vi"("error in (no error)"=w142, "refnum name"=w135, "CTRE_CANcoder_DeviceRef"=w143) -> ("error out"=w52:errorcluster, "CTRE_CANcoder_DeviceRef"=w51:T27)  [unwired: 7 in]
  n93 = Build Path(base path=w16, name or relative path=w8) -> (appended path=w9:path)
  "appended path" <- w9
  n94 = call-poly <vilib>:"Read Delimited Spreadsheet.vi"("file path (dialog if empty)"=w9) -> ("all rows"=w2:dbl[][], "error out"=w15:errorcluster)  [unwired: 9 in, 4 out]
  n95 = call <vilib>:"CTRE_Phoenix_CANcoder_SetStatusFrameRate.vi"("error in (no error)"=w52, "Period (ms)"=w53, "CANcoder Status Frame"=w54, "CTRE_CANcoder_DeviceRef"=w51) -> ("error out"=w44:errorcluster)  [unwired: 6 in, 1 out]
  n96 = call <vilib>:"CTRE_Phoenix_CANcoder_Open.vi"("error in"=w44, "Device Number"=u8 25) -> ("error out"=w140:errorcluster, "CTRE_CANcoder_DeviceRef"=w141:T27)  [unwired: 8 in]
  n97 = call <vilib>:"CTRE_Phoenix_CANcoder_RefNumRegistrySet.vi"("error in (no error)"=w140, "refnum name"=w134, "CTRE_CANcoder_DeviceRef"=w141) -> ("error out"=w42:errorcluster, "CTRE_CANcoder_DeviceRef"=w41:T27)  [unwired: 7 in]
  n98 = call <vilib>:"CTRE_Phoenix_CANcoder_SetStatusFrameRate.vi"("error in (no error)"=w42, "Period (ms)"=w50, "CANcoder Status Frame"=w49, "CTRE_CANcoder_DeviceRef"=w41) -> ("error out"=w43:errorcluster)  [unwired: 6 in, 1 out]
  n99 = call <vilib>:"CTRE_Phoenix_CANcoder_Open.vi"("error in"=w43, "Device Number"=u8 26) -> ("error out"=w138:errorcluster, "CTRE_CANcoder_DeviceRef"=w139:T27)  [unwired: 8 in]
  n100 = call <vilib>:"CTRE_Phoenix_CANcoder_RefNumRegistrySet.vi"("error in (no error)"=w138, "refnum name"=w133, "CTRE_CANcoder_DeviceRef"=w139) -> ("error out"=w39:errorcluster, "CTRE_CANcoder_DeviceRef"=w40:T27)  [unwired: 7 in]
  n101 = call <vilib>:"CTRE_Phoenix_CANcoder_SetStatusFrameRate.vi"("error in (no error)"=w39, "Period (ms)"=w47, "CANcoder Status Frame"=w48, "CTRE_CANcoder_DeviceRef"=w40) -> ("error out"=w36:errorcluster)  [unwired: 6 in, 1 out]
  n102 = call <vilib>:"CTRE_Phoenix_CANcoder_Open.vi"("error in"=w36, "Device Number"=u8 27) -> ("error out"=w136:errorcluster, "CTRE_CANcoder_DeviceRef"=w137:T27)  [unwired: 8 in]
  n103 = call <vilib>:"CTRE_Phoenix_CANcoder_RefNumRegistrySet.vi"("error in (no error)"=w136, "refnum name"=w132, "CTRE_CANcoder_DeviceRef"=w137) -> ("error out"=w37:errorcluster, "CTRE_CANcoder_DeviceRef"=w38:T27)  [unwired: 7 in]
  n104 = call <vilib>:"CTRE_Phoenix_CANcoder_SetStatusFrameRate.vi"("error in (no error)"=w37, "Period (ms)"=w46, "CANcoder Status Frame"=w45, "CTRE_CANcoder_DeviceRef"=w38) -> ("error out"=→"error out":errorcluster)  [unwired: 6 in, 1 out]
  n105 = Unbundle By Name(w15) -> ("status"=w7:bool)
  "File Read Error" <- w7
  n106 = Index Array(array=w2, index (col)=0 ("disabled index (col)")) -> (element=w13:dbl[])  [unwired: 1 in]
  n107 = Array Size(array=w13) -> (size(s)=w11:i32)
  "elements" <- w11
  n108 = Not(x=w7) -> (.not. x?=w6:bool)
  n109 = Equal?(x=w11, y=4) -> (x = y?=w10:bool)
  n110 = And(x=w10, y=w6) -> (x .and. y?=w3:bool)
  n111 = case shown="False" w3 {
    tunnel: w2 -> [_ w218]
    tunnel: w1 -> [w217 _]
    frame False {
      # "0th index alpha, 1st index beta"
      n112 = Index Array(array="Front_Left_Zero", index=w217) -> (element=w211:dbl)
      n113 = Index Array(array="Front_Right_Zero", index=w217) -> (element=w212:dbl)
      n114 = Index Array(array="Back_Left_Zero", index=w217) -> (element=w210:dbl)
      n115 = Index Array(array="Back_Right_Zero", index=w217) -> (element=w209:dbl)
      n116 = global write "Drive_Globals.vi" "Front_Right_Zero"(w212) -> ()
      n117 = global write "Drive_Globals.vi" "Front_Left_Zero"(w211) -> ()
      n118 = global write "Drive_Globals.vi" "Back_Right_Zero"(w209) -> ()
      n119 = global write "Drive_Globals.vi" "Back_Left_Zero"(w210) -> ()
    }
    frame True {
      n120 = for {
        tunnel: w218 -> [w222] mode=indexing
        i -> [w220]
        n121 = Index Array(array=w222, index=0) -> (element=w219:dbl)
        n122 = case shown="3" w220 {
          tunnel: w219 -> [w223 w224 w225 w226]
          frame 0, Default {
            n123 = global write "Drive_Globals.vi" "Front_Right_Zero"(w223) -> ()
          }
          frame 1 {
            n124 = global write "Drive_Globals.vi" "Front_Left_Zero"(w224) -> ()
          }
          frame 2 {
            n125 = global write "Drive_Globals.vi" "Back_Left_Zero"(w225) -> ()
          }
          frame 3 {
            n126 = global write "Drive_Globals.vi" "Back_Right_Zero"(w226) -> ()
          }
        }
      }
    }
  }
